vi "Get Vision Angle.vi"(1 "Camera Resolution (in pixels, along the axis you want)":dbl=640.0, 2 "Object Position (in pixels)":dbl, 3 "Camer FOV (in degrees)":dbl=65.0) -> (0 "Object Position (in degrees)":dbl)   [LabVIEW 2015]
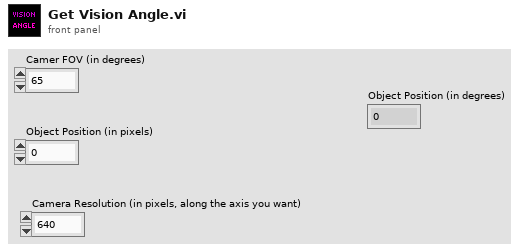
[diagram p1: front panel]
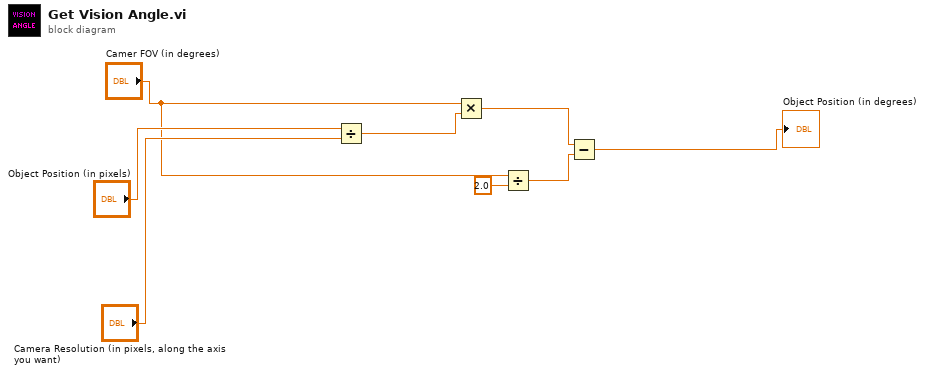
[diagram p0: block diagram]
diagram:
  n1 = Divide(x="Object Position (in pixels)", y="Camera Resolution (in pixels, along the axis you want)") -> (x/y=w6:dbl)
  n2 = Multiply(x="Camer FOV (in degrees)", y=w6) -> (x*y=w5:dbl)
  n3 = Divide(x="Camer FOV (in degrees)", y=2.0) -> (x/y=w2:dbl)
  n4 = Subtract(x=w5, y=w2) -> (x-y=→"Object Position (in degrees)":dbl)
